vi "mlink_enc_init.vi"(8 "error in (no error)":errorcluster, 9 "init value":i32, 10 "channel":u8, 11 "connection ID":i32=-1) -> (0 "error out":errorcluster, 3 "connection ID out":i32)   [LabVIEW 2009, in "MicroDAQ.lvlib" / "mlink.lvlib"]
doc: "This function initializes selected quadrature encoder module (ENC1, ENC2) with provided initial value. The function has to be called before mlink_enc_read() function call."
uses:
  <instrlib>/MicroDAQ/Mlink library wraper/mlink.lvlib
  <instrlib>/MicroDAQ/MLink32.dll
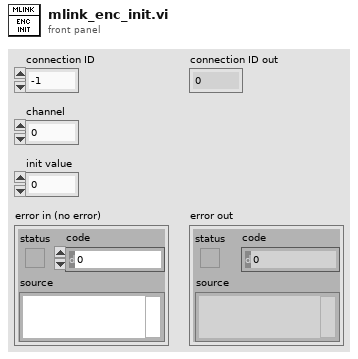
[diagram p1: front panel]
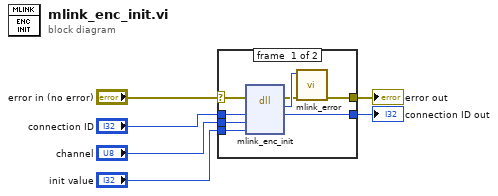
[diagram p0: block diagram]
diagram:
  n1 = case shown="No Error" "error in (no error)" {
    selector: "error in (no error)" -> [w12 w16]
    tunnel: "connection ID" -> [w14 w15]
    tunnel: [w13 w15] -> w5
    tunnel: [w9 w16] -> w3
    tunnel: "init value" -> [w8 _]
    tunnel: "channel" -> [w7 _]
    frame #0 {
      n2 = dll-call lib="C:/Program Files (x86)/National Instruments/LabVIEW 2009/instr.lib/MicroDAQ/MLink32.dll" fn="mlink_enc_init"(error in=w12, "connection ID"=w14, "channel"=w7, "init_value"=w8) -> (error out=w10:errorcluster, "return type"=w11:i32, "connection ID"=w13:i32)  [unwired: 4 in, 1 out]
      n3 = call <instrlib>:"mlink_error.vi"("error in (no error)"=w10, "error code"=w11) -> ("error out"=w9:errorcluster)  [unwired: 9 in]
    }
    frame #1 {
    }
  }
  "connection ID out" <- w5
  "error out" <- w3
